vi "FRCts20_Backend_FormErrorStatus.vi"(8 "error in (no error)":errorcluster) -> (0 "error out":errorcluster, 3 "String":string)   [LabVIEW 2014, in "FRCts20_Backend_Engine.lvlib"]
doc: "Takes an error and formats it into a string so that it can be received by any backend api accessors. Normally, it removes errors from the code stream so that the error-returning code can execute. However, in the case of a connection loss, we create a new error (9999) and pass that through."
uses:
  FRCts20_Backend_Engine.lvlib
  <vilib>/regexp/Match Regular Expression.xnode
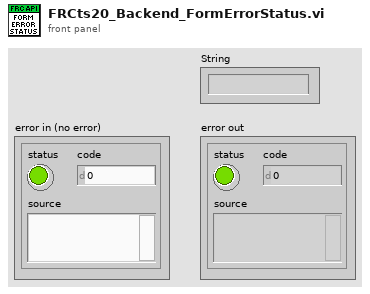
[diagram p1: front panel]
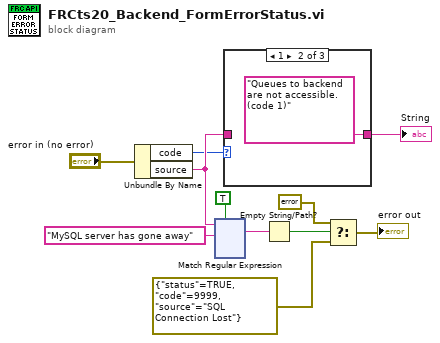
[diagram p0: block diagram]
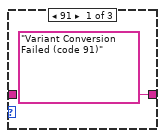
[diagram p2: hidden frame]
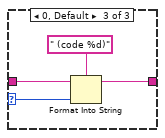
[diagram p3: hidden frame]
diagram:
  n1 = Unbundle By Name("error in (no error)") -> ("code"=w2:i32, "source"=w9:string)
  n2 = xnode "Match Regular Expression"("input string"=w9, "regular expression"="MySQL server has gone away", "ignore case? (F)"=TRUE) -> ("whole match"=w7:string)  [unwired: 3 in, 4 out]
  n3 = case shown="1" w2 {
    selector: w2 -> [_ _ w14]
    tunnel: ["Variant Conversion Failed (code 91)" "Queues to backend are not accessible. (code 1)" w16] -> w11
    tunnel: w9 -> [_ _ w15]
    frame 91 {
    }
    frame 1 {
    }
    frame 0, Default {
      n4 = Format Into String(format string=" (code %d)", initial string=w15, w14) -> (resulting string=w16:string)  [unwired: 1 in, 1 out]
    }
  }
  "String" <- w11
  n5 = Empty String/Path?(string/path=w7) -> (empty?=w6:bool)
  n6 = Select(t=errorcluster {"status"=FALSE, "code"=0, "source"=""}, s=w6, f=errorcluster {"status"=TRUE, "code"=9999, "source"="SQL Connection Lost"}) -> (s? t:f=→"error out":errorcluster)
